vi "fgv_status-display.vi"(7 "Mode":enum16{"Initial", "Update", "Clear"}(ring)=enum."Update", 8 "error in":errorcluster, 9 "detail":string, 10 "title":string, 11 "System Log":refnum<vi>) -> (0 "error out":errorcluster)   [LabVIEW 2021]
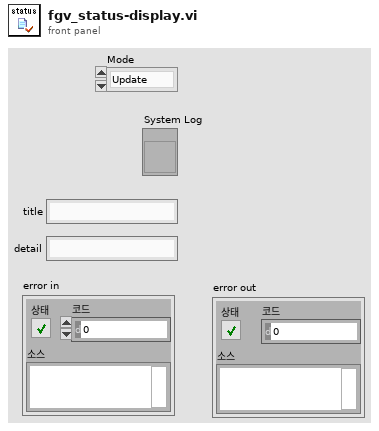
[diagram p1: front panel]
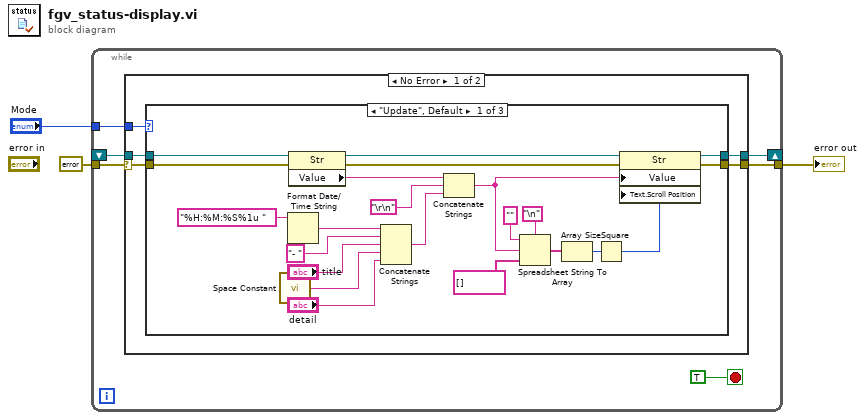
[diagram p0: block diagram]
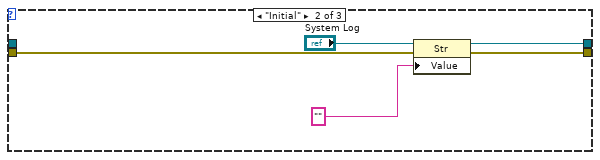
[diagram p2: hidden frame]
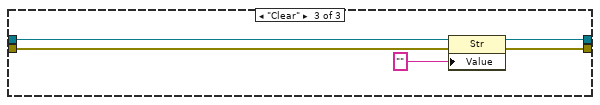
[diagram p3: hidden frame]
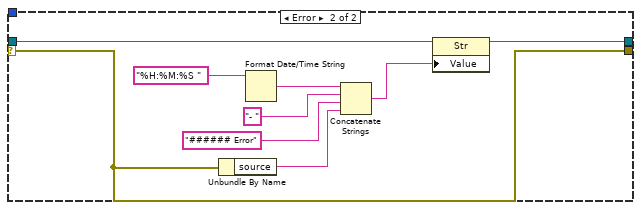
[diagram p4: hidden frame]
diagram:
  n1 = while {
    tunnel: errorcluster {"status"=FALSE, "code"=0, "source"=""} ("error in") -> [w4]
    tunnel: [w9] -> w3
    tunnel: "Mode" -> [w7]
    shift-right: [w6] -> _
    shift-left: _ -> [w5]
    stop <- TRUE stop-if-true
    n2 = case shown="No Error" w4 {
      selector: w4 -> [w10 w47]
      tunnel: [w14 w47] -> w9
      tunnel: w7 -> [w13 _]
      tunnel: [w12 w54] -> w6
      tunnel: w5 -> [w11 w55]
      frame No Error {
        n3 = case shown="\"Update\", Default" w13 {
          tunnel: w11 -> [w36 _ w44]
          tunnel: w10 -> [w31 w38 w46]
          tunnel: [w30 w39 w45] -> w14
          tunnel: [w29 w40 w43] -> w12
          frame "Update", Default {
            n4 = call <vilib>:"Space Constant.vi"() -> ("String"=w16:string)
            n5 = Format Date/Time String(time format string (%c)="%H:%M:%S%1u " ("시간 포맷 문자열 (%c)")) -> (date/time string=w21:string)  [unwired: 2 in]
            n6 = property class="Str"(reference=w36, error in=w31) -> (reference out=w33:refnum<vi>, error out=w32:errorcluster, "Value"=w35:string)
            n7 = Concatenate Strings(w21, "- " ("포맷 문자열"), "title", w16, "detail") -> (w20:string)
            n8 = Concatenate Strings(w35, "\r\n", w20) -> (w24:string)
            n9 = Spreadsheet String To Array(delimiter (Tab)="\n", format string="" ("포맷 문자열"), spreadsheet string=w24, array type (2D Dbl)=string[] []) -> (array=w28:string[])
            n10 = Array Size(array=w28) -> (size(s)=w23:i32)
            n11 = Square(x=w23) -> (x^2=w15:i32)
            n12 = property class="Str"(reference=w33, error in=w32, "Value"=w24, "Text.Scroll Position"=w15) -> (reference out=w29:refnum<vi>, error out=w30:errorcluster)
          }
          frame "Initial" {
            n13 = property class="Str"(reference="System Log", error in=w38, "Value"="" ("값")) -> (reference out=w40:refnum<vi>, error out=w39:errorcluster)
          }
          frame "Clear" {
            n14 = property class="Str"(reference=w44, error in=w46, "Value"="" ("값")) -> (reference out=w43:refnum<vi>, error out=w45:errorcluster)
          }
        }
      }
      frame Error {
        n15 = Unbundle By Name(w47) -> ("source"=w49:string)
        n16 = Format Date/Time String(time format string (%c)="%H:%M:%S " ("시간 포맷 문자열 (%c)")) -> (date/time string=w52:string)  [unwired: 2 in]
        n17 = Concatenate Strings(w52, "- " ("포맷 문자열"), "###### Error" ("문자열"), w49) -> (w50:string)
        n18 = property class="Str"(reference=w55, "Value"=w50) -> (reference out=w54:refnum<vi>)  [unwired: 1 in, 1 out]
      }
    }
  }
  "error out" <- w3
